vi "Replace file.vi"(8 "error in":errorcluster caption="error in (no error)", 9 "password":string, 10 "new wifi name":string, 11 "txt input":string) -> (0 "error out":errorcluster caption="error out (no error)", 3 "txt output":string)   [LabVIEW 2013]
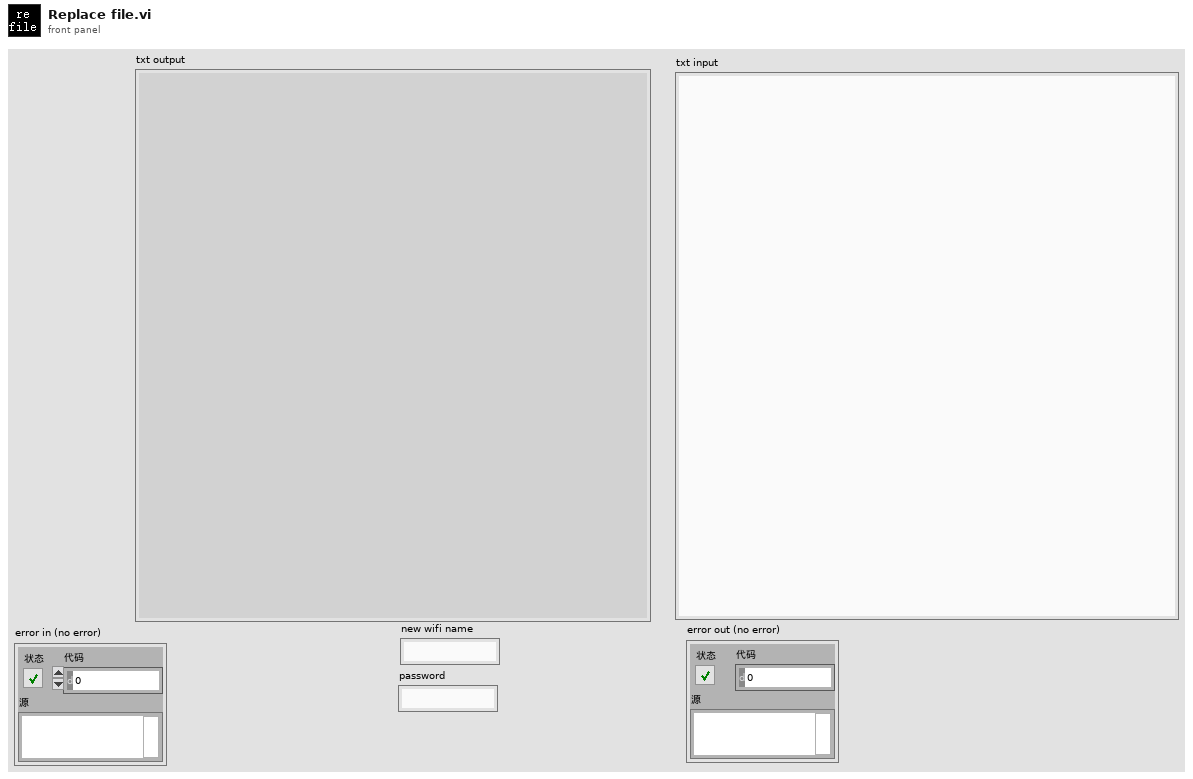
[diagram p1: front panel]
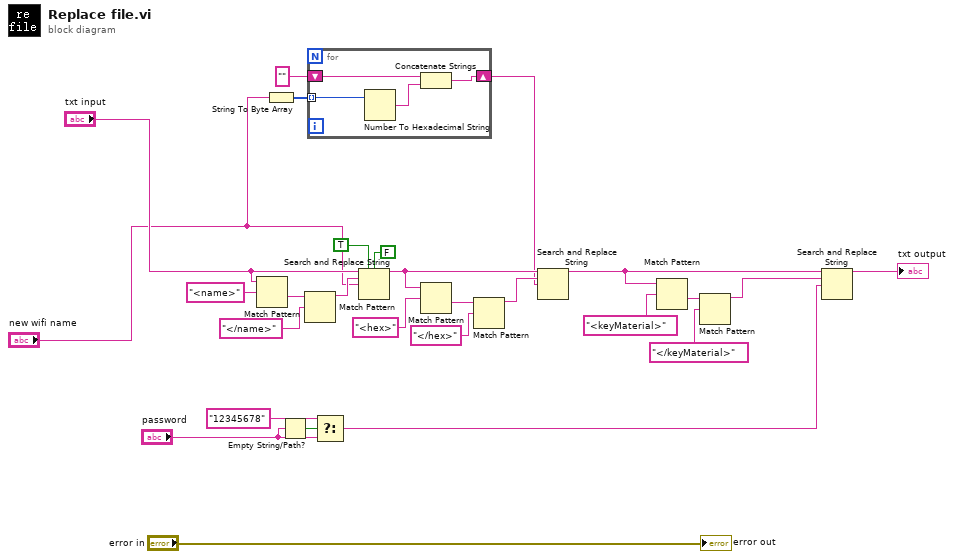
[diagram p0: block diagram]
diagram:
  n1 = Match Pattern(string="txt input", regular expression="<name>" ("正则表达式")) -> (after substring=w26:string)  [unwired: 1 in, 3 out]
  n2 = String To Byte Array(string="new wifi name") -> (unsigned byte array=w9:u8[])
  n3 = Empty String/Path?(string/path="password") -> (empty?=w4:bool)
  n4 = Match Pattern(string=w26, regular expression="</name>" ("正则表达式")) -> (before substring=w24:string)  [unwired: 1 in, 3 out]
  n5 = for {
    tunnel: w9 -> [w31] mode=indexing
    shift-right: [w28] -> w6
    shift-left: "" ("字符串") -> [w30]
    n6 = Number To Hexadecimal String(2:w31) -> (0:w29:string)  [unwired: 1 in]
    n7 = Concatenate Strings(w30, w29) -> (w28:string)
  }
  n8 = Select(t="12345678" ("正则表达式"), s=w4, f="password") -> (s? t:f=w1:string)
  n9 = Search and Replace String(replace all?=TRUE ("替换全部？(F)"), case sensitive?=FALSE ("忽略大小写？(F)"), input string="txt input", search string=w24, replace string="new wifi name") -> (result string=w20:string)  [unwired: 3 in, 3 out]
  n10 = Match Pattern(string=w20, regular expression="<hex>" ("正则表达式")) -> (after substring=w22:string)  [unwired: 1 in, 3 out]
  n11 = Match Pattern(string=w22, regular expression="</hex>" ("正则表达式")) -> (before substring=w19:string)  [unwired: 1 in, 3 out]
  n12 = Search and Replace String(input string=w20, search string=w19, replace string=w6) -> (result string=w10:string)  [unwired: 5 in, 3 out]
  n13 = Match Pattern(string=w10, regular expression="<keyMaterial>" ("正则表达式")) -> (after substring=w16:string)  [unwired: 1 in, 3 out]
  n14 = Match Pattern(string=w16, regular expression="</keyMaterial>" ("正则表达式")) -> (before substring=w15:string)  [unwired: 1 in, 3 out]
  n15 = Search and Replace String(input string=w10, search string=w15, replace string=w1) -> (result string=→"txt output":string)  [unwired: 5 in, 3 out]
  "error out" <- "error in"
